vi "set_sku.vi"(6 "timeout (25000ms)":i32=25000, 8 "error in (no error)":errorcluster, 9 "SKU ID":T1, 10 "sku hex filepath":path, 11 "daemon reference in":refnum<k5>) -> (0 "error out":errorcluster, 2 "response":string, 3 "daemon reference out":refnum<k5>, 5 "command out":string="random")   [LabVIEW 2017]
doc: "<b>Command: </b>\"set_sku\"\n\n<b>Description: </b> This command set sku config hexfile to device to allow ddm perform certain function in eol.\n\n<b>Parameters: </b> sku configuration hexfile, sku id\n____________________________________________\nDIPC 692 Daemon API 10.0.0.1\nSam Tee - Dyson Technology Ltd\nCopyright (c) 2024, Dyson Technology Ltd"
uses:
  typdef/sku_id.ctl
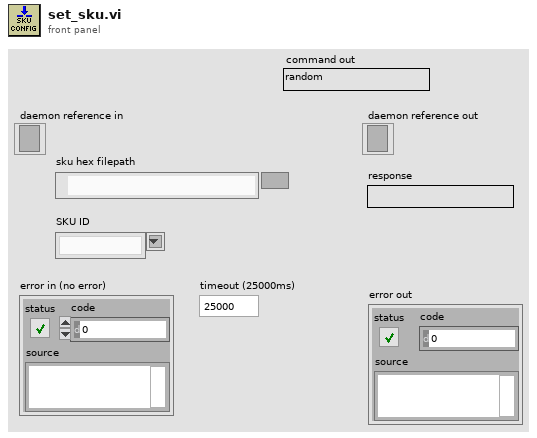
[diagram p1: front panel]
types:
  T1 = typedef "sku_id.ctl" = string
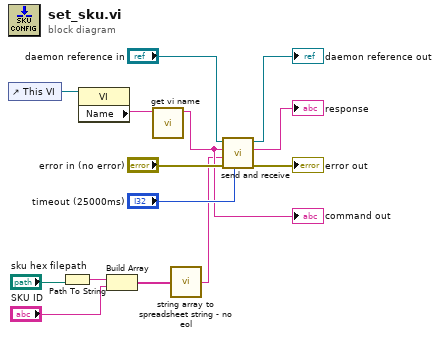
[diagram p0: block diagram]
diagram:
  n1 = control-ref of="This VI"() -> (w8:refnum<vi>)
  n2 = Path To String(path="sku hex filepath") -> (string=w4:string)
  n3 = property class="VI"(reference=w8) -> ("Name"=w7:string)  [unwired: 1 in, 2 out]
  n4 = Build Array(w4, "SKU ID") -> (w2:T1[])
  n5 = call "get vi name.vi"("library.lvlib:name.vi"=w7) -> ("vi name"=w6:string)  [unwired: 10 in]
  "command out" <- w6
  n6 = call "string array to spreadsheet string - no eol.vi"("string array"=w2) -> ("spreadsheet string - no eol"=w1:string)
  n7 = call "send and receive.vi"("timeout (25000ms)"="timeout (25000ms)", "error in (no error)"="error in (no error)", "data"=w1, "command"=w6, "daemon reference in"="daemon reference in") -> ("error out"=→"error out":errorcluster, "response"=→"response":string, "daemon reference out"=→"daemon reference out":refnum<k5>)  [unwired: 4 in]
